vi "Convert Voltage to Angle-with Caraya Assertions.vi"(10 "Inclinometer output (V)":dbl) -> (2 "Angle":dbl)   [LabVIEW 2018]
uses:
  <vilib>/addons/_JKI Toolkits/Caraya/classes/Assert/Assert.lvclass
panel:
  # "Run this VI to with different Inclinometer output values and see how \nthe assertion VIs generate an error if the voltage is not between\n0.5V and 4.5V."
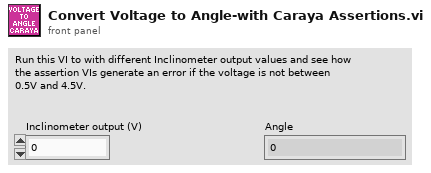
[diagram p1: front panel]
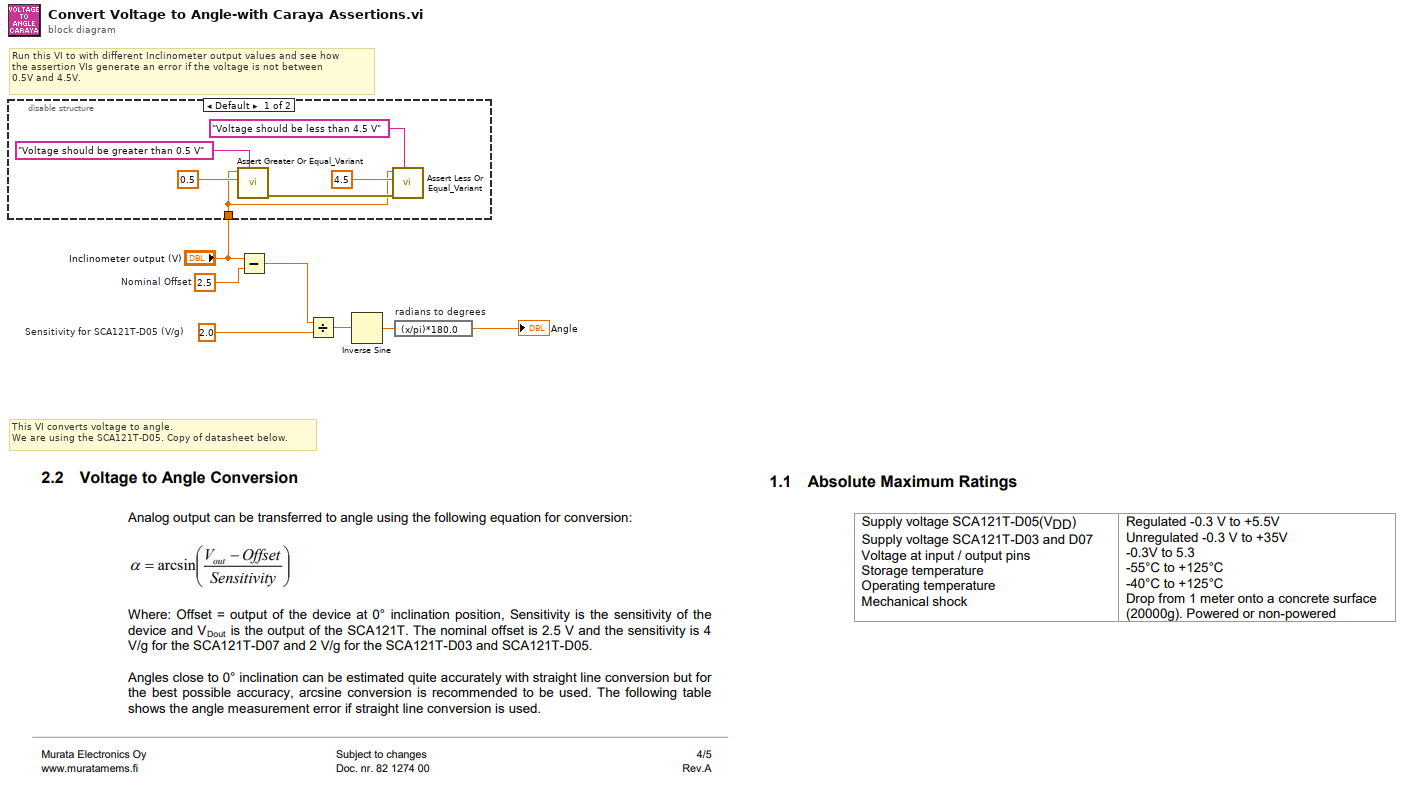
[diagram p0: block diagram]
diagram:
  w4 = 2.5  # Nominal Offset
  w6 = 2.0  # Sensitivity for SCA121T-D05 (V/g)
  # "Run this VI to with different Inclinometer output values and see how \nthe assertion VIs generate an error if the voltage is not between\n0.5V and 4.5V."
  # "This VI converts voltage to angle.\nWe are using the SCA121T-D05. Copy of datasheet below."
  n1 = disable-structure shown="Default" {
    disable-tunnel: "Inclinometer output (V)" -> [w10 _]
    frame condition #0 (active) {
      n2 = call <vilib>:"Assert Greater Or Equal_Variant.vi"("Label"="Voltage should be greater than 0.5 V", "Y"=0.5 ("Minimum voltage\n(equivalent to -90 degrees)"), "X"=w10) -> ("error out"=w12:errorcluster)  [unwired: 8 in]
      n3 = call <vilib>:"Assert Less Or Equal_Variant.vi"("Label"="Voltage should be less than 4.5 V", "error in (no error)"=w12, "Y"=4.5 ("Maximum voltage\n(equivalent to -90 degrees)"), "X"=w10) -> ()  [unwired: 7 in, 1 out]
    }
    frame condition #1 {
    }
  }
  n4 = Subtract(x="Inclinometer output (V)", y=w4) -> (x-y=w5:dbl)
  n5 = Divide(x=w5, y=w6) -> (x/y=w7:dbl)
  n6 = Inverse Sine(1:w7) -> (0:w3:dbl)
  n7 = expression code="(x/pi)*180.0" "radians to degrees"(w3) -> (→"Angle":dbl)
